vi "stringToDatetimeForStart.vi"(9 "input string":string) -> (1 "date/time string":string, 3 "sqltime string":string, 4 "Shift":string, 6 "ShiftDate":string)   [LabVIEW 2012]
uses:
  <vilib>/Utility/miscctls.llb/LVDateTimeRec.ctl
panel:
  in  "date time rec":T1
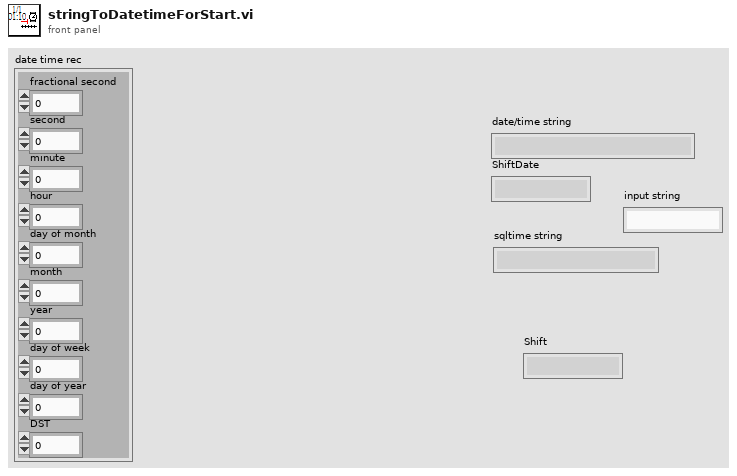
[diagram p1: front panel]
types:
  T1 = typedef "LVDateTimeRec.ctl" = cluster{"fractional second":dbl, "second":i32, "minute":i32, "hour":i32, "day of month":i32, "month":i32, "year":i32, "day of week":i32, "day of year":i32, "DST":i32}
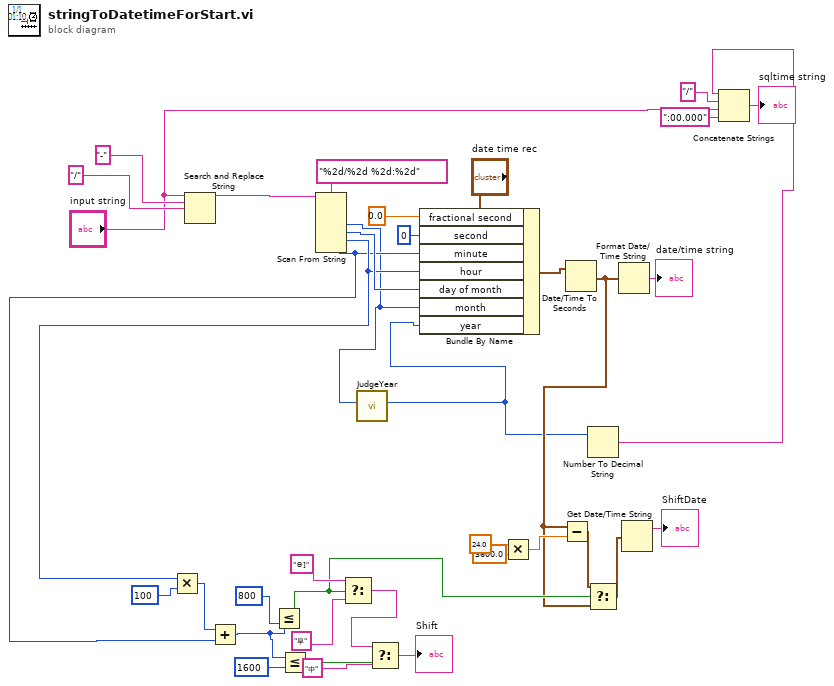
[diagram p0: block diagram]
diagram:
  n1 = Search and Replace String(input string="input string", search string="-", replace string="/" ("replace string (\"\")")) -> (result string=w29:string)  [unwired: 5 in, 3 out]
  n2 = Scan From String(format string="%2d/%2d %2d:%2d", input string=w29) -> (output 1=w2:i32, output 2=w33:i32, output 3=w13:i32, output 4=w12:i32)  [unwired: 6 in, 3 out]
  n3 = Multiply(x=w13, y=100) -> (x*y=w22:i32)
  n4 = Add(x=w22, y=w12) -> (x+y=w15:i32)
  n5 = Less Or Equal?(x=w15, y=800) -> (x <= y?=w6:bool)
  n6 = Less Or Equal?(x=w15, y=1600) -> (x <= y?=w17:bool)
  n7 = Select(t="©]", s=w6, f="早") -> (s? t:f=w14:string)
  n8 = call "JudgeYear.vi"("DataMonth"=w2) -> ("DataYear"=w1:i32)  [unwired: 10 in]
  n9 = Select(t=w14, s=w17, f="中") -> (s? t:f=→"Shift":string)
  n10 = Bundle By Name(cluster="date time rec", "fractional second"=0.0, "second"=0, "minute"=w12, "hour"=w13, "day of month"=w33, "month"=w2, "year"=w1) -> (w35:T1)
  n11 = Multiply(x=24.0, y=3600.0) -> (x*y=w9:dbl)
  n12 = Date/Time To Seconds(2:w35) -> (0:w4:timestamp)  [unwired: 1 in]
  n13 = Subtract(x=w4, y=w9) -> (x-y=w5:timestamp)
  n14 = Number To Decimal String(number=w1) -> (decimal integer string=w28:string)  [unwired: 1 in]
  n15 = Select(t=w5, s=w6, f=w4) -> (s? t:f=w3:timestamp)
  n16 = Format Date/Time String(seconds (now)=w4) -> (date/time string=→"date/time string":string)  [unwired: 2 in]
  n17 = Get Date/Time String(seconds (now)=w3) -> (date string=→"ShiftDate":string)  [unwired: 2 in, 1 out]
  n18 = Concatenate Strings(w28, "/" ("string"), "input string", ":00.000" ("string")) -> (→"sqltime string":string)
